vi "GdsLanguage_FindAllControls.vi"(0 "ViRef":refnum<vi>, 1 "LabelMatchPattern":string, 5 "error in (no error)":errorcluster) -> (15 "ControlsFound":refnum<vi>[](array[refnum]), 19 "error out":errorcluster)   [LabVIEW 2020]
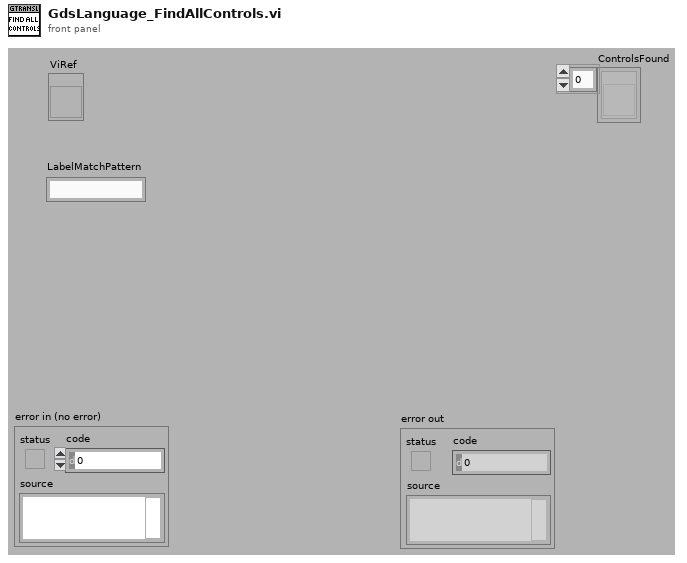
[diagram p1: front panel]
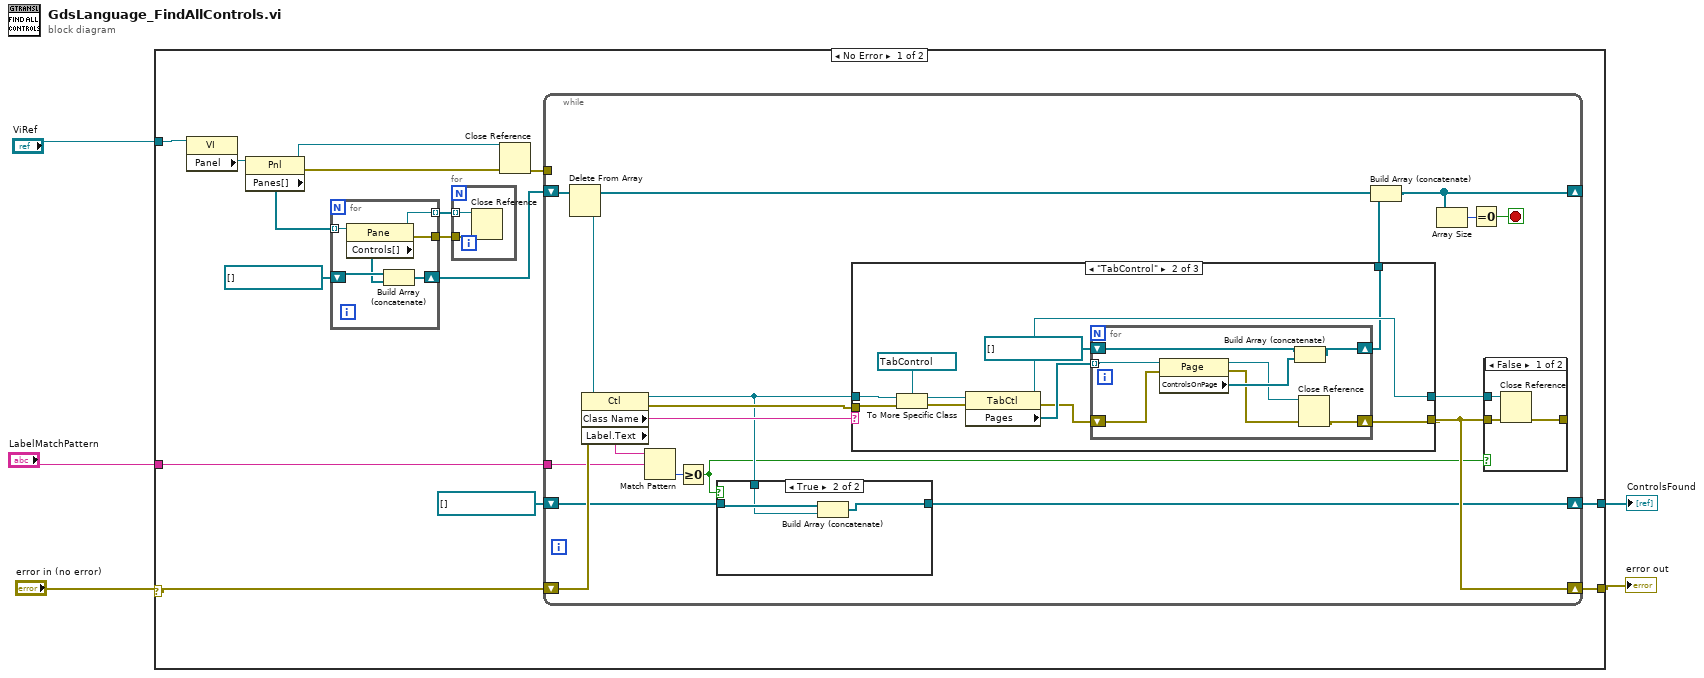
[diagram p0: block diagram]
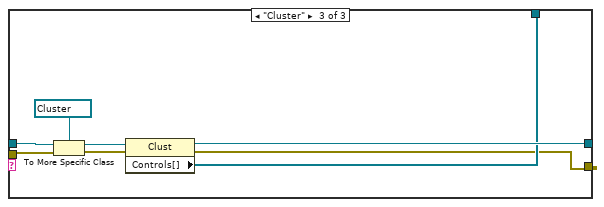
[diagram p5: hidden frame]
diagram:
  n1 = case shown="No Error" "error in (no error)" {
    selector: "error in (no error)" -> [w18 w84]
    tunnel: [w20 w84] -> w5
    tunnel: "ViRef" -> [w19 _]
    tunnel: [w17 _] -> w2
    tunnel: "LabelMatchPattern" -> [w12 _]
    frame No Error {
      n2 = property class="VI"(reference=w19) -> ("Panel"=w15:refnum<vi>)  [unwired: 1 in, 2 out]
      n3 = property class="Pnl"(reference=w15) -> (reference out=w16:refnum<vi>, error out=w14:errorcluster, "Panes[]"=w11:refnum<vi>[])  [unwired: 1 in]
      n4 = for {
        tunnel: w11 -> [w28] mode=indexing
        shift-right: [w27] -> w9
        shift-left: refnum<vi>[] [] -> [w26]
        tunnel: [w24] -> w8
        tunnel: [w23] -> w7 mode=indexing
        n5 = property class="Pane"(reference=w28) -> (reference out=w23:refnum<vi>, error out=w24:errorcluster, "Controls[]"=w25:refnum<vi>[])  [unwired: 1 in]
        n6 = Build Array (concatenate)(w26, w25) -> (w27:refnum<vi>[])
      }
      n7 = for {
        tunnel: w8 -> [w22]
        tunnel: w7 -> [w21] mode=indexing
        n8 = Close Reference(reference=w21, error in (no error)=w22) -> ()  [unwired: 1 out]
      }
      n9 = Close Reference(reference=w16, error in (no error)=w14) -> (error out=w6:errorcluster)
      n10 = while {
        shift-right: [w42] -> _
        shift-left: w9 -> [w47]
        shift-right: [w39] -> w20
        shift-left: w18 -> [w40]
        shift-right: [w31] -> w17
        shift-left: refnum<vi>[] [] -> [w32]
        tunnel: w12 -> [w34]
        tunnel: w6 -> [_]
        stop <- w45 stop-if-true
        n11 = Delete From Array(array=w47) -> (deleted portion=w38:refnum<vi>, array with subset deleted=w43:refnum<vi>[])  [unwired: 2 in]
        n12 = property class="Ctl"(reference=w38, error in=w40) -> (reference out=w30:refnum<vi>, error out=w44:errorcluster, "Class Name"=w37:string, "Label.Text"=w35:string)
        n13 = Match Pattern(string=w35, regular expression=w34) -> (offset past match=w33:i32)  [unwired: 1 in, 3 out]
        n14 = Greater Or Equal To 0?(x=w33) -> (x >= 0?=w29:bool)
        n15 = case shown="True" w29 {
          tunnel: w32 -> [w51 w54]
          tunnel: [w51 w53] -> w31
          tunnel: w30 -> [_ w52]
          frame False {
          }
          frame True {
            n16 = Build Array (concatenate)(w54, w52) -> (w53:refnum<vi>[])
          }
        }
        n17 = case shown="\"TabControl\"" w37 {
          tunnel: w30 -> [w56 w67 w83]
          tunnel: w44 -> [w55 w62 w79]
          tunnel: [w55 w60 w76] -> w39
          tunnel: [_ w58 w77] -> w36
          tunnel: [w56 w61 w78] -> w41
          frame Default {
          }
          frame "TabControl" {
            n18 = To More Specific Class(target class=refnum<vi> refnum ("CaseSelector"), reference=w67, error in=w62) -> (specific class reference=w65:refnum<vi>, error out=w63:errorcluster)
            n19 = property class="TabCtl"(reference=w65, error in=w63) -> (reference out=w61:refnum<vi>, error out=w59:errorcluster, "Pages"=w64:refnum<vi>[])
            n20 = for {
              tunnel: w64 -> [w75] mode=indexing
              shift-right: [w68] -> w60
              shift-left: w59 -> [w74]
              shift-right: [w71] -> w58
              shift-left: refnum<vi>[] [] -> [w73]
              n21 = property class="Page"(reference=w75, error in=w74) -> (reference out=w69:refnum<vi>, error out=w70:errorcluster, "ControlsOnPage"=w72:refnum<vi>[])
              n22 = Build Array (concatenate)(w73, w72) -> (w71:refnum<vi>[])
              n23 = Close Reference(reference=w69, error in (no error)=w70) -> (error out=w68:errorcluster)
            }
          }
          frame "Cluster" {
            n24 = To More Specific Class(target class=refnum<vi> refnum ("CaseSelector"), reference=w83, error in=w79) -> (specific class reference=w81:refnum<vi>, error out=w80:errorcluster)
            n25 = property class="Clust"(reference=w81, error in=w80) -> (reference out=w78:refnum<vi>, error out=w76:errorcluster, "Controls[]"=w77:refnum<vi>[])
          }
        }
        n26 = Build Array (concatenate)(w43, w36) -> (w42:refnum<vi>[])
        n27 = Array Size(array=w42) -> (size(s)=w46:i32)
        n28 = Equal To 0?(x=w46) -> (x = 0?=w45:bool)
        n29 = case shown="False" w29 {
          tunnel: w41 -> [w50 _]
          tunnel: w39 -> [w49 _]
          tunnel: [w48 _] -> _
          frame False {
            n30 = Close Reference(reference=w50, error in (no error)=w49) -> (error out=w48:errorcluster)
          }
          frame True {
          }
        }
      }
    }
    frame Error {
    }
  }
  "error out" <- w5
  "ControlsFound" <- w2
